vi "Utility MXA-PXA Wait for OPC.vi"(5 "Wait (s)":dbl=90.0 format="%#_13g", 6 "Error In":errorcluster, 9 "VISA Resource In":refnum<visa-resource-name>="PSA1") -> (0 "Error Out":errorcluster, 1 "Aborted?":bool, 2 "OPC?":bool, 3 "VISA Resource Out":refnum<visa-resource-name>)   [LabVIEW 2014]
panel:
  out "Elapsed (s)":dbl
  in  "Stop":bool
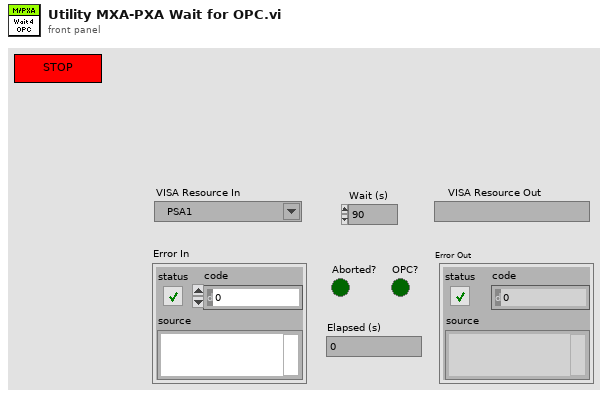
[diagram p1: front panel]
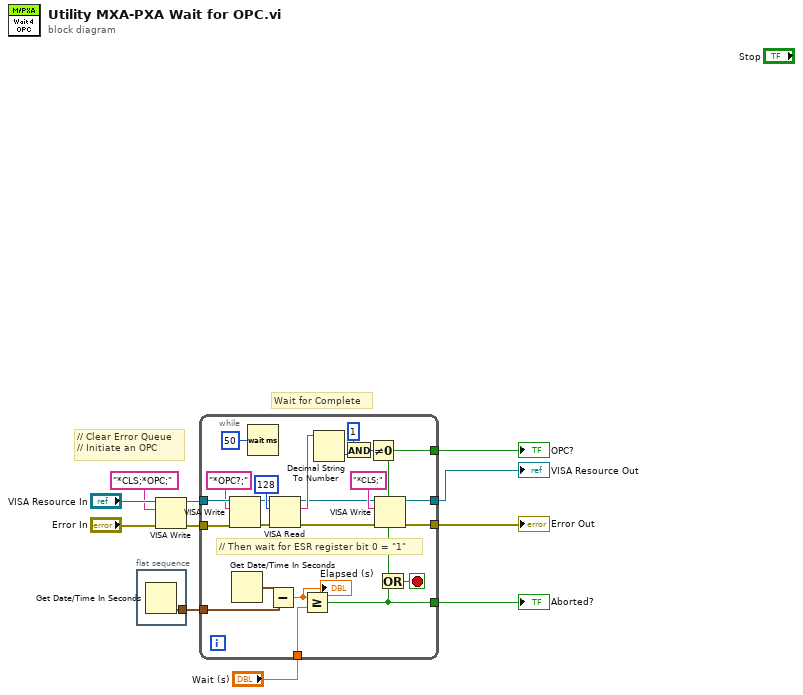
[diagram p0: block diagram]
diagram:
  # "// Clear Error Queue\n// Initiate an OPC"
  # "Wait for Complete"
  n1 = flat-sequence {
    tunnel: [w12] -> w11
    frame #0 {
      n2 = Get Date/Time In Seconds() -> (seconds since 1Jan1904=w12:timestamp)
    }
  }
  n3 = VISA Write(VISA resource name="VISA Resource In", write buffer="*CLS;*OPC;", error in (no error)="Error In") -> (VISA resource name out=w6:refnum<visa-resource-name>, error out=w4:errorcluster)  [unwired: 1 out]
  n4 = while {
    tunnel: w4 -> [w35]
    tunnel: w6 -> [w34]
    tunnel: w11 -> [w23]
    tunnel: [w21] -> w10
    tunnel: "Wait (s)" -> [w20]
    tunnel: [w13] -> w2
    tunnel: [w19] -> w8
    tunnel: [w15] -> w1
    stop <- w24 stop-if-true
    # "// Then wait for ESR register bit 0 = \"1\""
    n5 = VISA Write(VISA resource name=w34, write buffer="*OPC?;", error in (no error)=w35) -> (VISA resource name out=w31:refnum<visa-resource-name>, error out=w32:errorcluster)  [unwired: 1 out]
    n6 = Get Date/Time In Seconds() -> (seconds since 1Jan1904=w28:timestamp)
    n7 = Wait (ms)(milliseconds to wait=u32 50 ("Wait (ms)")) -> ()  [unwired: 1 out]
    n8 = Subtract(x=w28, y=w23) -> (x-y=w27:dbl)
    "Elapsed (s)" <- w27
    n9 = VISA Read(VISA resource name=w31, byte count=u32 128, error in (no error)=w32) -> (VISA resource name out=w14:refnum<visa-resource-name>, read buffer=w18:string, error out=w16:errorcluster)  [unwired: 1 out]
    n10 = Greater Or Equal?(x=w27, y=w20) -> (x >= y?=w21:bool)
    n11 = Decimal String To Number(string=w18) -> (number=w30:i32)  [unwired: 2 in, 1 out]
    n12 = And(x=1, y=w30) -> (x .and. y?=w26:i32)
    n13 = Not Equal To 0?(x=w26) -> (x != 0?=w19:bool)
    n14 = VISA Write(VISA resource name=w14, write buffer="*CLS;", error in (no error)=w16) -> (VISA resource name out=w13:refnum<visa-resource-name>, error out=w15:errorcluster)  [unwired: 1 out]
    n15 = Or(x=w19, y=w21) -> (x .or. y?=w24:bool)
  }
  "Error Out" <- w1
  "Aborted?" <- w10
  "VISA Resource Out" <- w2
  "OPC?" <- w8
